vi "InitFromXML.vi"(8 "error in (no error)":errorcluster, 10 "XML":string, 11 "Manual in":refnum<class "Manual.lvclass">) -> (0 "error out":errorcluster, 3 "Manual out":refnum<class "Manual.lvclass">)   [LabVIEW 2009, in "NavScreen.lvlib" / "Manual.lvclass"]
uses:
  Manual.lvclass
  ClickableText/ClickableText.lvclass
  Manual.lvclass/Manual.ctl
  NavScreen.lvlib
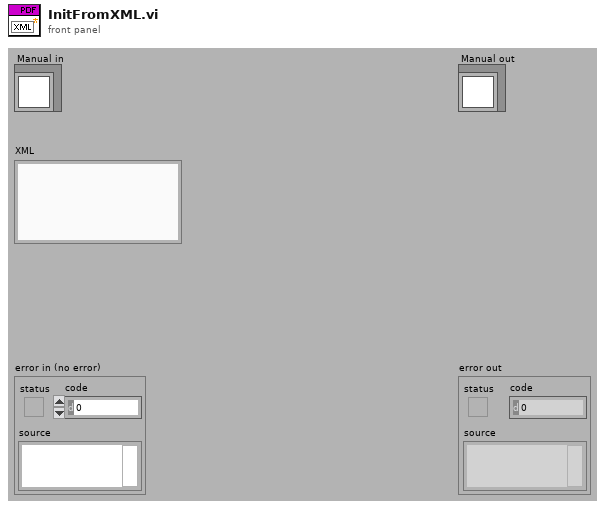
[diagram p1: front panel]
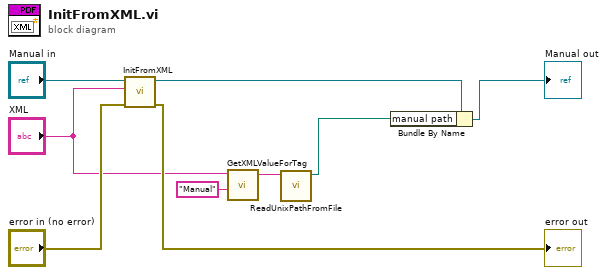
[diagram p0: block diagram]
diagram:
  n1 = call-parent "InitFromXML.vi"("error in (no error)"="error in (no error)", "XML"="XML", "ClickableText in"="Manual in") -> ("error out"=→"error out":errorcluster, "ClickableText out"=w6:refnum<class "Manual.lvclass">)  [unwired: 7 in]
  n2 = call "GetXMLValueForTag.vi"("tag"="Manual", "XML"="XML") -> ("value"=w2:string)  [unwired: 8 in, 1 out]
  n3 = call "ReadUnixPathFromFile.vi"("path"=w2) -> ("path"=w1:path)  [unwired: 10 in]
  n4 = Bundle By Name(cluster=w6, "manual path"=w1) -> (→"Manual out":refnum<class "Manual.lvclass">)
